vi "MIO Get Fake QCurve.vi"(1 "Lower Limit":dbl format="%.2f", 2 "Upper Limit":dbl format="%.2f", 3 "Sweeps":i32) -> (0 "Waveform Graph":dbl[](graph))   [LabVIEW 2009]
uses:
  QCA Global.vi
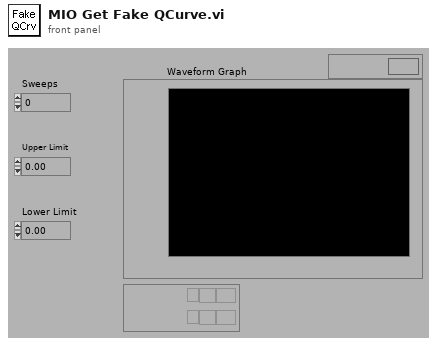
[diagram p1: front panel]
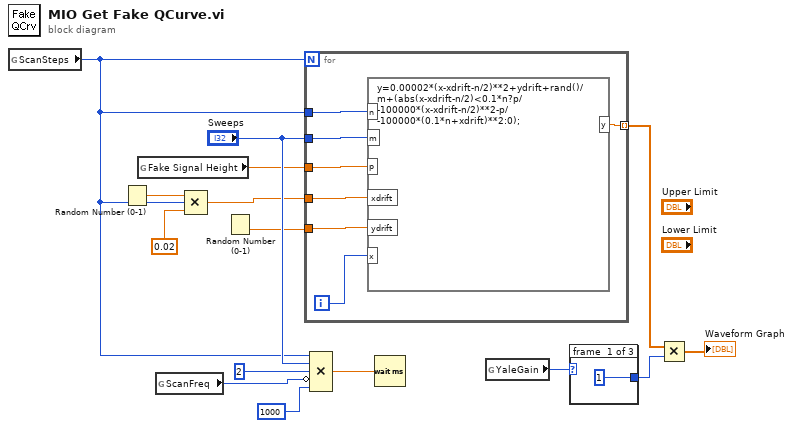
[diagram p0: block diagram]
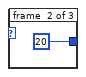
[diagram p2: hidden frame]
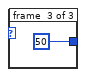
[diagram p3: hidden frame]
diagram:
  n1 = global read "QCA Global.vi" "ScanSteps"() -> (w10:i32)
  n2 = Random Number (0-1)() -> (number: 0 to 1=w13:dbl)
  n3 = global read "QCA Global.vi" "Fake Signal Height"() -> (w14:dbl)
  n4 = global read "QCA Global.vi" "ScanFreq"() -> (w7:i32)
  n5 = Compound Arithmetic op=MULTIPLY(w13, w10, 0.02) -> (w11:dbl)
  n6 = Random Number (0-1)() -> (number: 0 to 1=w12:dbl)
  n7 = for {
    N: w10 -> [_]
    tunnel: w10 -> [w22]
    tunnel: "Sweeps" -> [w21]
    tunnel: [w20] -> w2 mode=indexing
    tunnel: w14 -> [w18]
    tunnel: w11 -> [w17]
    tunnel: w12 -> [w16]
    i -> [w19]
    n8 = formula code="y=0.00002*(x-xdrift-n/2)**2+ydrift+rand()/m+(abs(x-xdrift-n/2)<0.1*n?p/-100000*(x-xdrift-n/2)**2-p/-100000*(0.1*n+xdrift)**2:0);"("x"=w19, "n"=w22, "m"=w21, "p"=w18, "xdrift"=w17, "ydrift"=w16) -> ("y"=w20:dbl)
  }
  n9 = Compound Arithmetic op=MULTIPLY(w10, "Sweeps", 2 ("Input"), invert w7, 1000) -> (w6:dbl)
  n10 = Wait (ms)(milliseconds to wait=w6) -> ()  [unwired: 1 out]
  n11 = global read "QCA Global.vi" "YaleGain"() -> (w4:i32)
  n12 = case shown="0, Default" w4 {
    tunnel: [1 20 50] -> w3
    frame #0 {
    }
    frame #1 {
    }
    frame #2 {
    }
  }
  n13 = Multiply(x=w2, y=w3) -> (x*y=→"Waveform Graph":dbl[])
